vi "Word cmd backup.vi"(6 "Word cmd":T3, 8 "Error In (no error)":errorcluster, 10 "Mathcad Output":T1, 11 "DesignRequest":T2) -> (0 "error out":errorcluster, 1 "Find-Replace":cluster{"Find":string, "Replace":string}[](array[cluster]), 4 "design spec  file path":path)   [LabVIEW 2011]
uses:
  Design Server.lvlib
  Folders.ctl
  Word cmd.ctl
  Variable cluster.ctl
  Design Request.ctl
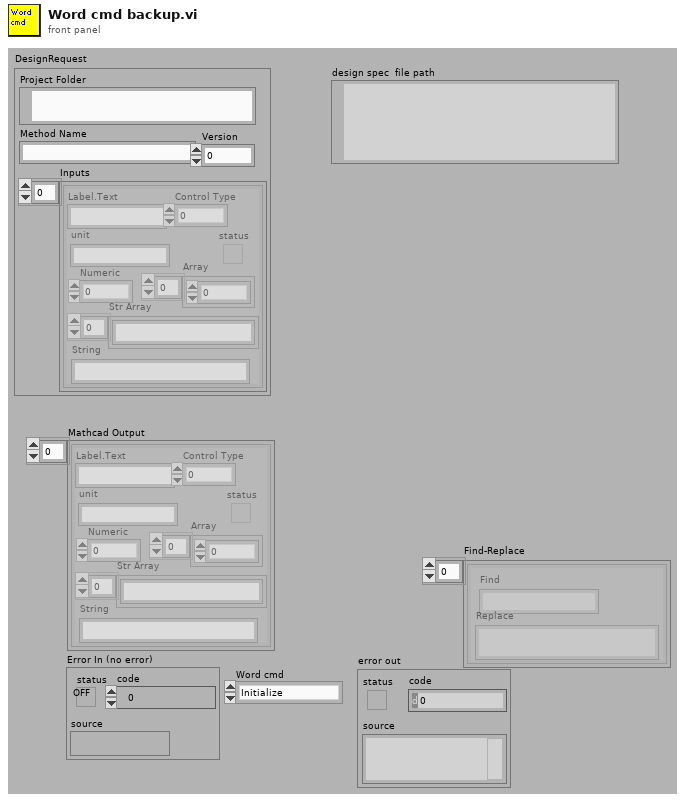
[diagram p1: front panel]
types:
  T1 = typedef "Design Server.lvlib/Variable cluster.ctl" = cluster{"Label.Text":string, "Control Type":u32, "Numeric":dbl, "Array":dbl[], "status":bool, "Str Array":string[], "String":string, "unit":string}[]
  T2 = typedef "Design Server.lvlib/Design Request.ctl" = cluster{"Project Folder":path, "Method Name":string, "Inputs":T1, "Version":i32}
  T3 = typedef "Design Server.lvlib/Word cmd.ctl" = enum16{"Initialize", "Create Reports", "Quit"}
  T4 = typedef "Design Server.lvlib/Folders.ctl" = enum16{"MathcadMethods", "RequestedDesigns", "CompletedDesigns", "MathcadCode", "CollabnetSVN.exe"}
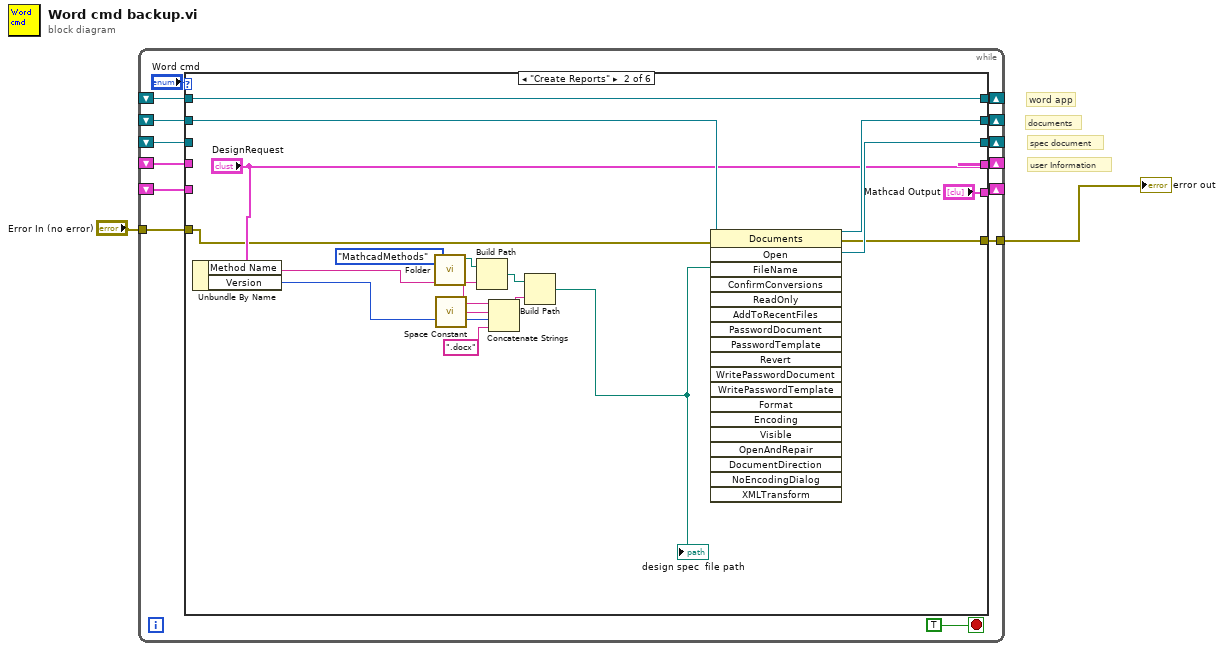
[diagram p0: block diagram]
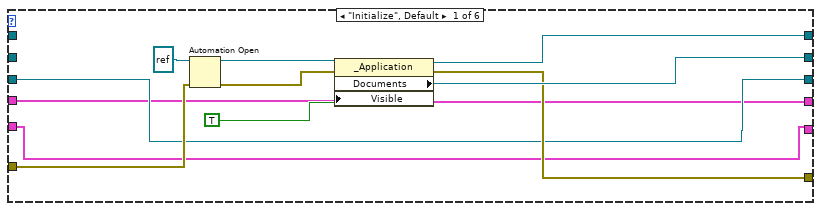
[diagram p2: hidden frame]
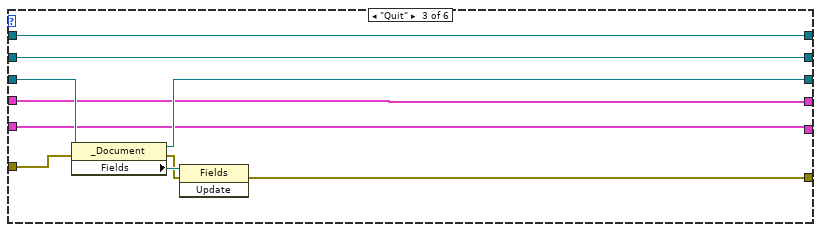
[diagram p3: hidden frame]
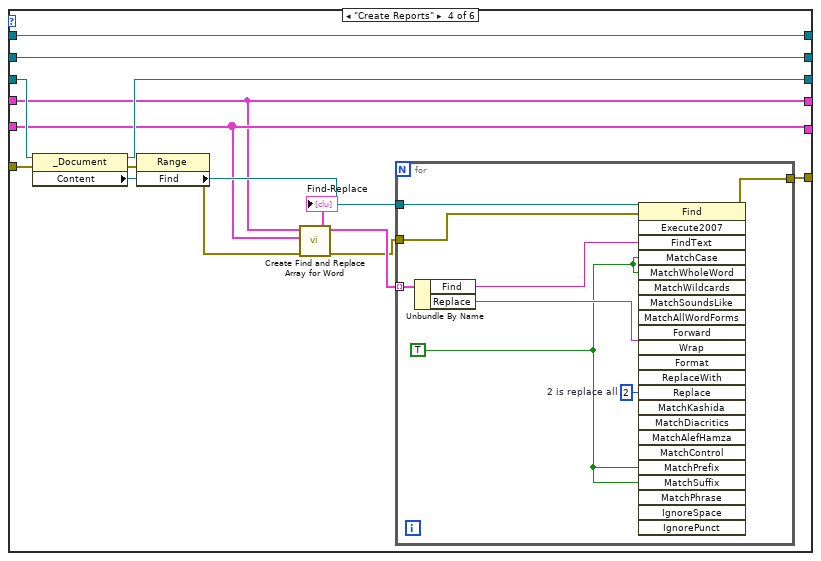
[diagram p4: hidden frame]
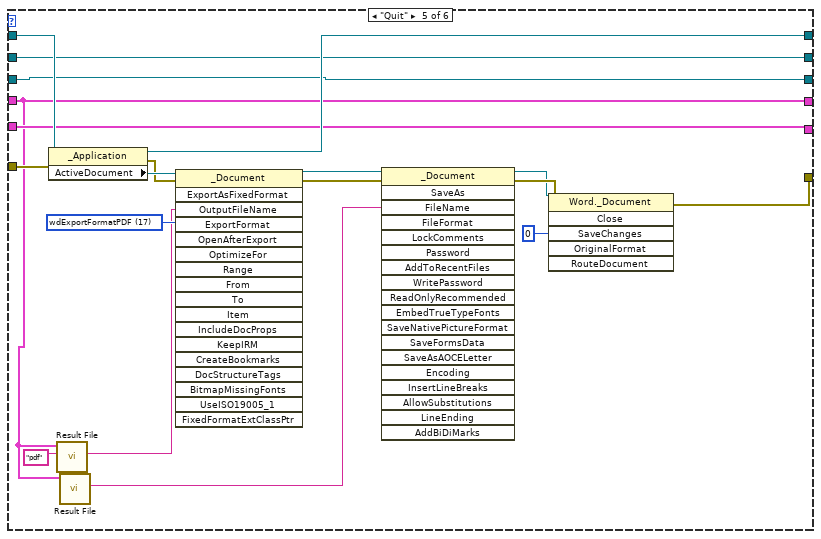
[diagram p5: hidden frame]
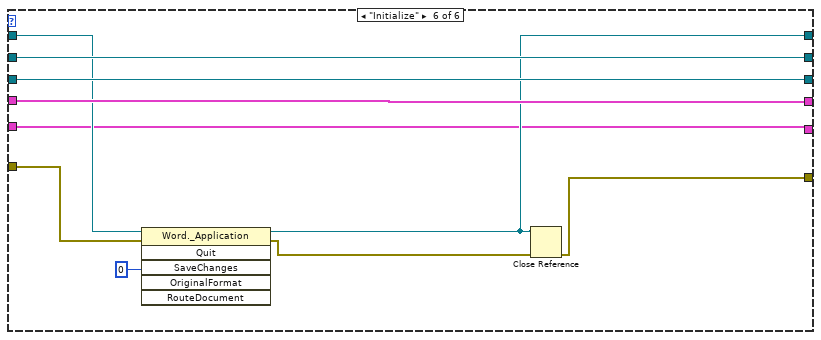
[diagram p6: hidden frame]
diagram:
  # "user Information"
  # "spec document"
  # "documents"
  # "word app"
  n1 = while {
    shift-right: [w14] -> _
    shift-left: _ -> [w9]
    shift-right: [w13] -> _
    shift-left: _ -> [w10]
    shift-right: [w12] -> _
    shift-left: _ -> [w11]
    tunnel: "Error In (no error)" -> [w8]
    tunnel: [w7] -> w1
    shift-right: [w6] -> _
    shift-left: _ -> [w5]
    shift-right: [w4] -> _
    shift-left: _ -> [w3]
    stop <- TRUE stop-if-true
    n2 = case shown="\"Create Reports\"" "Word cmd" {
      tunnel: [w23 w44 w50 w68 w90 w100] -> w14
      tunnel: [w22 w42 w51 w67 w89 w105] -> w13
      tunnel: [w19 w41 w52 w62 w88 w104] -> w12
      tunnel: w11 -> [w19 _ w54 w63 w88 w104]
      tunnel: w10 -> [_ w43 w51 w67 w89 w105]
      tunnel: w9 -> [_ w44 w50 w68 w92 w102]
      tunnel: w8 -> [w21 w28 w49 w61 w91 w99]
      tunnel: [w20 w40 w47 w60 w86 w97] -> w7
      tunnel: [w18 "DesignRequest" w46 w55 w78 w103] -> w6
      tunnel: w5 -> [w18 _ w46 w55 w78 w103]
      tunnel: [w17 "Mathcad Output" w45 w56 w81 w96] -> w4
      tunnel: w3 -> [w17 _ w45 w56 w81 w96]
      frame "Initialize", Default {
        n3 = Automation Open(error in (no error)=w21, Automation Refnum=refnum<k7> refnum ("Word._Application")) -> (Automation Refnum=w27:refnum<k7>, error out=w26:errorcluster)  [unwired: 2 in]
        n4 = property class="_Application"(reference=w27, error in=w26, "Visible"=TRUE) -> (reference out=w23:refnum<k7>, error out=w20:errorcluster, "Documents"=w22:refnum<k7>)
      }
      frame "Create Reports" {
        n5 = Unbundle By Name("DesignRequest") -> ("Method Name"=w32:string, "Version"=w29:i32)
        n6 = call "Folder.vi"("Folders"=Folders."MathcadMethods") -> ("FolderPath"=w36:path)  [unwired: 8 in, 2 out]
        n7 = call <vilib>:"Space Constant.vi"() -> ("String"=w33:string)
        n8 = Build Path(base path=w36, name or relative path=w32) -> (appended path=w35:path)
        n9 = Concatenate Strings(w32, w33, w29, ".docx" ("string")) -> (w34:string)
        n10 = Build Path(base path=w35, name or relative path=w34) -> (appended path=w30:path)
        "design spec  file path" <- w30
        n11 = invoke class="Documents" method="Open"(reference=w43, error in=w28, "FileName"=w30) -> (reference out=w42:refnum<k7>, error out=w40:errorcluster, "Open"=w41:refnum<k7>)  [unwired: 16 in, 16 out]
      }
      frame "Quit" {
        n12 = property class="_Document"(reference=w54, error in=w49) -> (reference out=w52:refnum<k7>, error out=w48:errorcluster, "Fields"=w53:refnum<k7>)
        n13 = invoke class="Fields" method="Update"(reference=w53, error in=w48) -> (error out=w47:errorcluster)  [unwired: 1 in, 2 out]
      }
      frame "Create Reports" {
        n14 = property class="_Document"(reference=w63, error in=w61) -> (reference out=w62:refnum<k7>, error out=w64:errorcluster, "Content"=w65:refnum<k7>)
        n15 = property class="Range"(reference=w65, error in=w64) -> (error out=w58:errorcluster, "Find"=w66:refnum<k7>)  [unwired: 1 out]
        n16 = call "Create Find and Replace Array for Word.vi"("error in"=w58, "Mathcad Output"=w56, "DesignRequest"=w55) -> ("error out"=w57:errorcluster, "Find-Replace"=w59:cluster{"Find":string, "Replace":string}[])  [unwired: 7 in]
        "Find-Replace" <- w59
        n17 = for {
          tunnel: w66 -> [w76]
          tunnel: w57 -> [w75]
          tunnel: [w73] -> w60
          tunnel: w59 -> [w72] mode=indexing
          w69 = TRUE ("Visible")
          w74 = 2  # 2 is replace all
          n18 = Unbundle By Name(w72) -> ("Find"=w71:string, "Replace"=w70:string)
          n19 = invoke class="Find" method="Execute2007"(reference=w76, error in=w75, "FindText"=w71, "MatchCase"=w69, "MatchWholeWord"=w69, "ReplaceWith"=w70, "Replace"=w74, "MatchPrefix"=w69, "MatchSuffix"=w69) -> (error out=w73:errorcluster)  [unwired: 14 in, 22 out]
        }
      }
      frame "Quit" {
        w93 = 17 items=["wdExportFormatPDF"=17, "wdExportFormatXPS"=18] ("ExportFormat")
        n20 = property class="_Application"(reference=w92, error in=w91) -> (reference out=w90:refnum<k7>, error out=w94:errorcluster, "ActiveDocument"=w95:refnum<k7>)
        n21 = call "Result File.vi"("File Type"="pdf", "DesignRequest"=w78) -> ("File string"=w79:string)  [unwired: 8 in, 1 out]
        n22 = call "Result File.vi"("DesignRequest"=w78) -> ("File string"=w77:string)  [unwired: 9 in, 1 out]
        n23 = invoke class="_Document" method="ExportAsFixedFormat"(reference=w95, error in=w94, "OutputFileName"=w79, "ExportFormat"=w93) -> (reference out=w83:refnum<k7>, error out=w85:errorcluster)  [unwired: 14 in, 16 out]
        n24 = invoke class="_Document" method="SaveAs"(reference=w83, error in=w85, "FileName"=w77) -> (reference out=w82:refnum<k7>, error out=w84:errorcluster)  [unwired: 16 in, 17 out]
        n25 = invoke class="Word._Document" method="Close"(reference=w82, error in=w84, "SaveChanges"=0) -> (error out=w86:errorcluster)  [unwired: 3 in, 5 out]
      }
      frame "Initialize" {
        n26 = invoke class="Word._Application" method="Quit"(reference=w102, error in=w99, "SaveChanges"=0) -> (reference out=w100:refnum<k7>, error out=w98:errorcluster)  [unwired: 3 in, 4 out]
        n27 = Close Reference(reference=w100, error in (no error)=w98) -> (error out=w97:errorcluster)
      }
    }
  }
  "error out" <- w1
